vi "抓邊_new.vi"(0 "Image In":T7, 1 "Process":T10(ring), 2 "Optimized Mode":bool, 5 "ROI":T8, 7 "Options":T6={"Search Direction"=0, "Edge Options"={"Edge Polarity"=0, "Kernel Size"=3, "Width"=3, "Minimum Edge Strength"=10.0, "Interpolation Type"=enum."Bilinear Fixed", "Data Processing Method"=enum."Average"}, "Show Search Area"=FALSE, "Show Search Lines"=FALSE, "Show Edges Found"=FALSE, "Show Result"=TRUE, "Search Area Color"=65280, "Search Lines Color"=255, "Edge Locations Color"=16776960, "Result Color"=16711680, "Overlay Group Name"=""} {"Edge Options"."Edge Polarity" items=["All Edges", "Rising Edges", "Falling Edges"]; "Edge Options"."Minimum Edge Strength" format="%.2f"; "Edge Options"."Width" step=2; "Edge Options"."Kernel Size" step=2; "Search Direction" items=["Left to Right", "Right to Left", "Top to Bottom", "Bottom to Top"]}, 9 "Gap":i32=10 min=1 max=300, 11 "error In":errorcluster, 13 "Point Diameter (5)":u32=5 min=3 max=1000) -> (4 "Image Out":T7, 6 "Line Profile":T9(graph), 8 "Line Segment":T1 {"Point 2"."Y" format="%.2f"; "Point 2"."X" format="%.2f"; "Point 1"."Y" format="%.2f"; "Point 1"."X" format="%.2f"}, 10 "Gradient Information":dbl[][](graph), 14 "Line Data":cluster{"X":sgl, "Y":sgl, "T":sgl}, 15 "error out":errorcluster)   [LabVIEW 2015]
uses:
  <vilib>/vision/Image Controls.llb/IMAQ Image.ctl
  <vilib>/vision/Measure.llb/Edge Options.ctl
  <vilib>/vision/Measure.llb/Edge Polarity.ctl
  <vilib>/vision/Measure.llb/Straight Edge Options.ctl
  <vilib>/vision/Measure.llb/Straight Edge Process.ctl
  <vilib>/vision/NI_Vision_Development_Module.lvlib
panel:
  in  "Line Fit Options":T2={"Number of Lines"=1, "Type"=enum."First Edge Rake", "Min. Score"=10.0, "Max. Score"=1000.0, "Orientation"=0.0, "Angle Range"=45.0, "Angle Tolerance"=1.0, "Step Size"=7, "Min. SNR (db)"=0.0, "Min. Points (%)"=25.0, "Hough Iterations"=5} {"Min. Points (%)" min=0.0 max=100.0; "Min. SNR (db)" min=0.0; "Max. Score" min=0.0 max=1024.0; "Min. Score" min=0.0 max=1024.0 step=1.0}
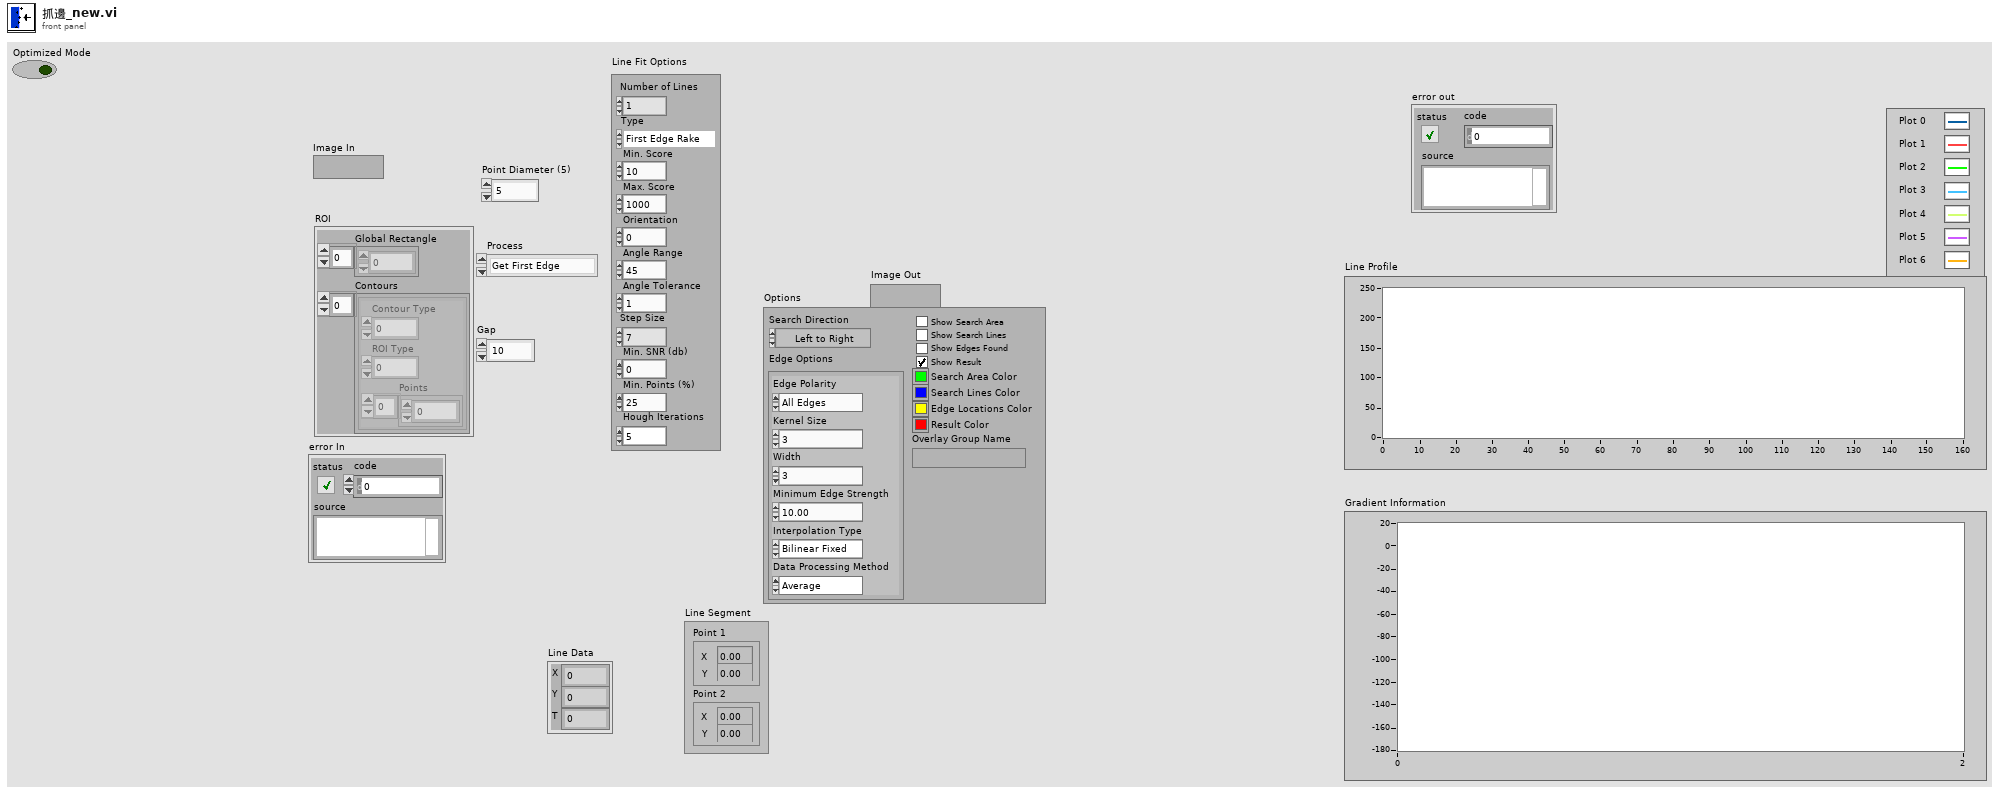
[diagram p1: front panel]
types:
  T1 = cluster{"Point 1":cluster{"X":sgl, "Y":sgl}, "Point 2":cluster{"X":sgl, "Y":sgl}}
  T2 = typedef "Straight Edge Options.ctl" = cluster{"Number of Lines":i32, "Type":T3, "Min. Score":dbl, "Max. Score":dbl, "Orientation":dbl, "Angle Range":dbl, "Angle Tolerance":dbl, "Step Size":u32, "Min. SNR (db)":dbl, "Min. Points (%)":dbl, "Hough Iterations":i32}
  T3 = typedef "Straight Edge Process.ctl" = enum32{"First Edge Rake", "Best Edge Rake", "Hough Edge Rake", "First Edge Projection", "Best Edge Projection"}
  T4 = typedef "Edge Options.ctl" = cluster{"Edge Polarity":T5, "Kernel Size":u32, "Width":u32, "Minimum Edge Strength":sgl, "Interpolation Type":enum32{"Zero Order", "Bilinear", "Quadratic", "Cubic", "Bilinear Fixed"}, "Data Processing Method":enum32{"Average", "Median"}}
  T5 = typedef "Edge Polarity.ctl" = u32
  T6 = cluster{"Search Direction":u32, "Edge Options":T4, "Show Search Area":bool, "Show Search Lines":bool, "Show Edges Found":bool, "Show Result":bool, "Search Area Color":u32, "Search Lines Color":u32, "Edge Locations Color":u32, "Result Color":u32, "Overlay Group Name":string}
  T7 = typedef "IMAQ Image.ctl" = refnum<image>
  T8 = cluster{"Global Rectangle":i32[], "Contours":cluster{"Contour Type":u32, "ROI Type":u32, "Points":i32[]}[]}
  T9 = cluster{"x0":sgl, "dx":sgl, "Pixels Line":sgl[]}[]
  T10 = enum16{"Get First Edge", "Get First + Last Edge", "Get All Edges", "Get Best Edge"}
  T11 = typedef "IMAQ Line" = cluster{"Start X":i32, "Start Y":i32, "End X":i32, "End Y":i32}
  T12 = cluster{"Point 1":cluster{"x":dbl, "y":dbl}, "Point 2":cluster{"x":dbl, "y":dbl}}
  T13 = typedef "IMAQ Rectangle" = cluster{"Left":i32, "Top":i32, "Right":i32, "Bottom":i32, "Rotation":dbl}
  T14 = typedef "IMAQ Point" = cluster{"X":sgl, "Y":sgl}
  T15 = cluster{"Left":i32, "Top":i32, "Right":i32, "Bottom":i32}
  T16 = typedef "ROI Descriptor" = cluster{"Global Rectangle":i32[], "Contours":cluster{"ID":enum32{"External", "Internal"}, "Type":u32, "Coordinates":i32[]}[]}
  T17 = typedef "Edge New.ctl" = cluster{"Location (Pixel)":cluster{"X":sgl, "Y":sgl}, "Location (Real-World)":cluster{"X":sgl, "Y":sgl}, "Distance (Pixel)":dbl, "Distance (Real-World)":dbl, "Strength":dbl, "Noise":dbl, "Rising?":bool}
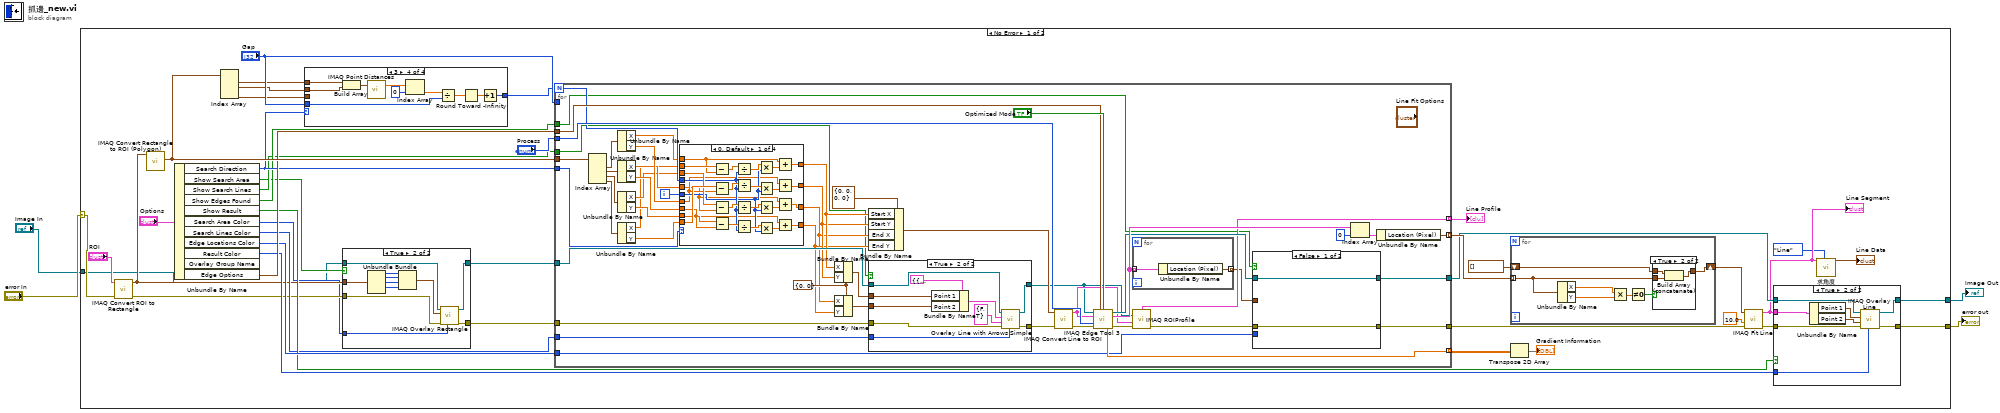
[diagram p0: block diagram]
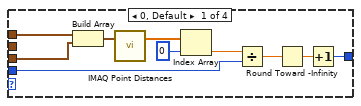
[diagram p4: hidden frame]
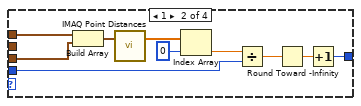
[diagram p5: hidden frame]
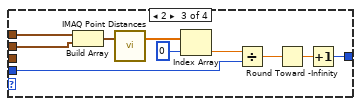
[diagram p6: hidden frame]
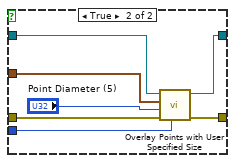
[diagram p9: hidden frame]
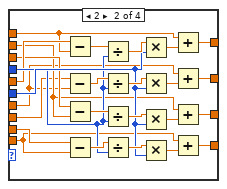
[diagram p10: hidden frame]
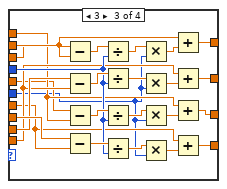
[diagram p11: hidden frame]
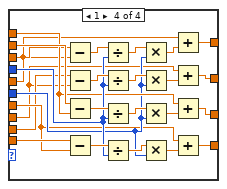
[diagram p12: hidden frame]
diagram:
  n1 = case shown="No Error" "error In" {
    selector: "error In" -> [w7 w297]
    tunnel: [w8 w297] -> w4
    tunnel: [w6 w296] -> w2
    tunnel: "Image In" -> [w5 w296]
    frame No Error {
      n2 = call "IMAQ Convert ROI to Rectangle"("error in (no error)"=w7, "ROI Descriptor"="ROI") -> ("error out"=w12:errorcluster, "Rectangle"=w13:T13)  [unwired: 7 in]
      n3 = call "IMAQ Convert Rectangle to ROI (Polygon)"("Rectangle"=w13) -> ("Rectangle Points"=w34:T14[])  [unwired: 7 in, 2 out]
      n4 = Unbundle By Name("Options") -> ("Search Direction"=w21:u32, "Show Search Area"=w10:bool, "Show Search Lines"=w16:bool, "Show Edges Found"=w19:bool, "Show Result"=w18:bool, "Search Area Color"=w9:u32, "Search Lines Color"=w15:u32, "Edge Locations Color"=w20:u32, "Result Color"=w17:u32, "Edge Options"=w22:T4)  [unwired: 1 out]
      n5 = Index Array(array=w34) -> (element #1=w32:T14, element #2=w31:T14, element #4=w30:T14)  [unwired: 4 in, 1 out]
      n6 = case shown="3" w21 {
        tunnel: "Gap" -> [w75 w85 w95 w105]
        tunnel: [w74 w84 w94 w104] -> w40
        tunnel: w32 -> [w71 w81 w93 w101]
        tunnel: w30 -> [w70 w80 _ _]
        tunnel: w31 -> [_ _ w89 w100]
        frame 0, Default {
          n7 = Build Array(w71, w70) -> (w73:T14[])
          n8 = call "IMAQ Point Distances"("Points"=w73) -> ("Distances"=w72:sgl[])  [unwired: 4 in, 1 out]
          n9 = Index Array(array=w72, index=0) -> (element=w68:sgl)
          n10 = Divide(x=w68, y=w75) -> (x/y=w76:sgl)
          n11 = Round Toward -Infinity(1:w76) -> (0:w77:sgl)
          n12 = Increment(x=w77) -> (x+1=w74:i32)
        }
        frame 1 {
          n13 = Build Array(w81, w80) -> (w83:T14[])
          n14 = call "IMAQ Point Distances"("Points"=w83) -> ("Distances"=w82:sgl[])  [unwired: 4 in, 1 out]
          n15 = Index Array(array=w82, index=0) -> (element=w78:sgl)
          n16 = Divide(x=w78, y=w85) -> (x/y=w86:sgl)
          n17 = Round Toward -Infinity(1:w86) -> (0:w87:sgl)
          n18 = Increment(x=w87) -> (x+1=w84:i32)
        }
        frame 2 {
          n19 = Build Array(w93, w89) -> (w92:T14[])
          n20 = call "IMAQ Point Distances"("Points"=w92) -> ("Distances"=w91:sgl[])  [unwired: 4 in, 1 out]
          n21 = Index Array(array=w91, index=0) -> (element=w90:sgl)
          n22 = Divide(x=w90, y=w95) -> (x/y=w96:sgl)
          n23 = Round Toward -Infinity(1:w96) -> (0:w97:sgl)
          n24 = Increment(x=w97) -> (x+1=w94:i32)
        }
        frame 3 {
          n25 = Build Array(w101, w100) -> (w103:T14[])
          n26 = call "IMAQ Point Distances"("Points"=w103) -> ("Distances"=w102:sgl[])  [unwired: 4 in, 1 out]
          n27 = Index Array(array=w102, index=0) -> (element=w99:sgl)
          n28 = Divide(x=w99, y=w105) -> (x/y=w106:sgl)
          n29 = Round Toward -Infinity(1:w106) -> (0:w107:sgl)
          n30 = Increment(x=w107) -> (x+1=w104:i32)
        }
      }
      n31 = case shown="True" w10 {
        tunnel: w5 -> [w45 w57]
        tunnel: [w45 w56] -> w14
        tunnel: w13 -> [_ w55]
        tunnel: w12 -> [w46 w49]
        tunnel: [w46 w48] -> w11
        tunnel: w9 -> [_ w47]
        frame False {
        }
        frame True {
          n32 = Unbundle(w55) -> ("Left"=w54:i32, "Top"=w53:i32, "Right"=w52:i32, "Bottom"=w51:i32)  [unwired: 1 out]
          n33 = Bundle("Left"=w54, "Top"=w53, "Right"=w52, "Bottom"=w51) -> (w50:T15)  [unwired: 1 in]
          n34 = call "IMAQ Overlay Rectangle"("Color"=w47, "error in (no error)"=w49, "Rectangle"=w50, "Image"=w57) -> ("error out"=w48:errorcluster, "Image Out"=w56:T7)  [unwired: 6 in]
        }
      }
      n35 = for {
        N: w40 -> [w154]
        tunnel: w21 -> [w152]
        tunnel: [w163] -> w37
        tunnel: w14 -> [w153]
        tunnel: w11 -> [w151]
        tunnel: [w162] -> w35
        tunnel: "Process" -> [w164]
        tunnel: w22 -> [w161]
        tunnel: [w160] -> w39 mode=indexing
        tunnel: [w159] -> w41 mode=indexing
        tunnel: [w158] -> w38 mode=indexing
        tunnel: "Gap" -> [_]
        tunnel: w34 -> [w150]
        tunnel: w20 -> [w122]
        tunnel: w19 -> [w121]
        tunnel: w16 -> [w120]
        tunnel: w15 -> [w119]
        i -> [w123]
        w147 = cluster{"X":i32, "Y":i32} {"X"=0, "Y"=0} ("Start Point")
        n36 = Index Array(array=w150) -> (element #1=w135:T14, element #2=w134:T14, element #3=w133:T14, element #4=w132:T14)  [unwired: 4 in]
        n37 = Unbundle By Name(w135) -> ("X"=w131:sgl, "Y"=w130:sgl)
        n38 = Unbundle By Name(w134) -> ("X"=w129:sgl, "Y"=w128:sgl)
        n39 = Unbundle By Name(w133) -> ("X"=w127:sgl, "Y"=w126:sgl)
        n40 = Unbundle By Name(w132) -> ("X"=w125:sgl, "Y"=w124:sgl)
        n41 = case shown="0, Default" w152 {
          tunnel: [w200 w219 w245 w270] -> w142
          tunnel: [w195 w218 w244 w271] -> w139
          tunnel: [w198 w216 w242 w268] -> w141
          tunnel: [w194 w217 w243 w269] -> w140
          tunnel: w125 -> [w213 w224 w250 w280]
          tunnel: w131 -> [w191 w226 w249 w279]
          tunnel: w154 -> [w204 w228 w255 w281]
          tunnel: w123 -> [w203 w229 w246 w278]
          tunnel: w124 -> [w210 w220 w252 w275]
          tunnel: w130 -> [w193 w222 w251 w274]
          tunnel: w127 -> [w207 w225 w248 w277]
          tunnel: w129 -> [w192 w227 w247 w276]
          tunnel: w126 -> [w202 w221 w253 w273]
          tunnel: w128 -> [w190 w223 w254 w272]
          frame 0, Default {
            n42 = Subtract(x=w213, y=w191) -> (x-y=w214:sgl)
            n43 = Subtract(x=w210, y=w193) -> (x-y=w212:sgl)
            n44 = Subtract(x=w207, y=w192) -> (x-y=w209:sgl)
            n45 = Subtract(x=w202, y=w190) -> (x-y=w205:sgl)
            n46 = Divide(x=w214, y=w204) -> (x/y=w215:sgl)
            n47 = Divide(x=w212, y=w204) -> (x/y=w211:sgl)
            n48 = Divide(x=w209, y=w204) -> (x/y=w208:sgl)
            n49 = Divide(x=w205, y=w204) -> (x/y=w206:sgl)
            n50 = Multiply(x=w215, y=w203) -> (x*y=w201:sgl)
            n51 = Multiply(x=w211, y=w203) -> (x*y=w199:sgl)
            n52 = Multiply(x=w208, y=w203) -> (x*y=w197:sgl)
            n53 = Multiply(x=w206, y=w203) -> (x*y=w196:sgl)
            n54 = Add(x=w191, y=w201) -> (x+y=w200:sgl)
            n55 = Add(x=w193, y=w199) -> (x+y=w198:sgl)
            n56 = Add(x=w192, y=w197) -> (x+y=w195:sgl)
            n57 = Add(x=w190, y=w196) -> (x+y=w194:sgl)
          }
          frame 2 {
            n58 = Subtract(x=w227, y=w226) -> (x-y=w240:sgl)
            n59 = Subtract(x=w223, y=w222) -> (x-y=w239:sgl)
            n60 = Subtract(x=w225, y=w224) -> (x-y=w237:sgl)
            n61 = Subtract(x=w221, y=w220) -> (x-y=w234:sgl)
            n62 = Divide(x=w240, y=w228) -> (x/y=w241:sgl)
            n63 = Divide(x=w239, y=w228) -> (x/y=w238:sgl)
            n64 = Divide(x=w237, y=w228) -> (x/y=w236:sgl)
            n65 = Divide(x=w234, y=w228) -> (x/y=w235:sgl)
            n66 = Multiply(x=w241, y=w229) -> (x*y=w233:sgl)
            n67 = Multiply(x=w238, y=w229) -> (x*y=w232:sgl)
            n68 = Multiply(x=w236, y=w229) -> (x*y=w231:sgl)
            n69 = Multiply(x=w235, y=w229) -> (x*y=w230:sgl)
            n70 = Add(x=w226, y=w233) -> (x+y=w219:sgl)
            n71 = Add(x=w222, y=w232) -> (x+y=w216:sgl)
            n72 = Add(x=w224, y=w231) -> (x+y=w218:sgl)
            n73 = Add(x=w220, y=w230) -> (x+y=w217:sgl)
          }
          frame 3 {
            n74 = Subtract(x=w248, y=w250) -> (x-y=w263:sgl)
            n75 = Subtract(x=w253, y=w252) -> (x-y=w260:sgl)
            n76 = Subtract(x=w247, y=w249) -> (x-y=w266:sgl)
            n77 = Subtract(x=w254, y=w251) -> (x-y=w265:sgl)
            n78 = Divide(x=w263, y=w255) -> (x/y=w262:sgl)
            n79 = Divide(x=w260, y=w255) -> (x/y=w261:sgl)
            n80 = Divide(x=w266, y=w255) -> (x/y=w267:sgl)
            n81 = Divide(x=w265, y=w255) -> (x/y=w264:sgl)
            n82 = Multiply(x=w262, y=w246) -> (x*y=w257:sgl)
            n83 = Multiply(x=w261, y=w246) -> (x*y=w256:sgl)
            n84 = Multiply(x=w267, y=w246) -> (x*y=w259:sgl)
            n85 = Multiply(x=w264, y=w246) -> (x*y=w258:sgl)
            n86 = Add(x=w250, y=w257) -> (x+y=w245:sgl)
            n87 = Add(x=w252, y=w256) -> (x+y=w242:sgl)
            n88 = Add(x=w249, y=w259) -> (x+y=w244:sgl)
            n89 = Add(x=w251, y=w258) -> (x+y=w243:sgl)
          }
          frame 1 {
            n90 = Subtract(x=w277, y=w276) -> (x-y=w289:sgl)
            n91 = Subtract(x=w273, y=w272) -> (x-y=w286:sgl)
            n92 = Subtract(x=w280, y=w279) -> (x-y=w292:sgl)
            n93 = Subtract(x=w275, y=w274) -> (x-y=w291:sgl)
            n94 = Divide(x=w289, y=w281) -> (x/y=w288:sgl)
            n95 = Divide(x=w286, y=w281) -> (x/y=w287:sgl)
            n96 = Divide(x=w292, y=w281) -> (x/y=w293:sgl)
            n97 = Divide(x=w291, y=w281) -> (x/y=w290:sgl)
            n98 = Multiply(x=w288, y=w278) -> (x*y=w283:sgl)
            n99 = Multiply(x=w287, y=w278) -> (x*y=w282:sgl)
            n100 = Multiply(x=w293, y=w278) -> (x*y=w285:sgl)
            n101 = Multiply(x=w290, y=w278) -> (x*y=w284:sgl)
            n102 = Add(x=w276, y=w283) -> (x+y=w270:sgl)
            n103 = Add(x=w272, y=w282) -> (x+y=w268:sgl)
            n104 = Add(x=w279, y=w285) -> (x+y=w271:sgl)
            n105 = Add(x=w274, y=w284) -> (x+y=w269:sgl)
          }
        }
        n106 = Bundle By Name(cluster=w147, "X"=w142, "Y"=w141) -> (w145:cluster{"X":i32, "Y":i32})
        n107 = Bundle By Name(cluster=w147, "X"=w139, "Y"=w140) -> (w146:cluster{"X":i32, "Y":i32})
        n108 = Bundle By Name(cluster=T11 {"Start X"=0, "Start Y"=0, "End X"=0, "End Y"=0} ("Line"), "Start X"=w142, "Start Y"=w141, "End X"=w139, "End Y"=w140) -> (w148:T11)
        n109 = case shown="True" w120 {
          tunnel: w153 -> [w170 w180]
          tunnel: w151 -> [w169 w179]
          tunnel: w146 -> [_ w178]
          tunnel: w145 -> [_ w177]
          tunnel: [w170 w173] -> w144
          tunnel: [w169 w172] -> w143
          tunnel: w119 -> [_ w171]
          frame False {
          }
          frame True {
            n110 = Bundle By Name(cluster=T12 {"Point 1"={"x"=50.0, "y"=50.0}, "Point 2"={"x"=70.0, "y"=70.0}} ("Line Coordinates"), "Point 1"=w177, "Point 2"=w178) -> (w174:T12)
            n111 = call "Overlay Line with Arrows Simple.vi"("Color"=w171, "error in"=w179, "Arrows"=cluster{"Start point":bool, "End point":bool} {"Start point"=FALSE, "End point"=TRUE}, "Line Coordinates"=w174, "Image In"=w180) -> ("error out"=w172:errorcluster, "Image Out"=w173:T7)  [unwired: 5 in]
          }
        }
        n112 = call "IMAQ Convert Line to ROI"("error in (no error)"=w143, "Line"=w148) -> ("error out"=w156:errorcluster, "ROI Descriptor"=w155:T16)  [unwired: 7 in]
        n113 = call "IMAQ Edge Tool 3"("Image"=w144, "Edge Options"=w161, "Optimized Mode"="Optimized Mode", "ROI Descriptor"=w155, "Process"=w164, "error in (no error)"=w156) -> ("Image (duplicate)"=w165:T7, "Edge Information"=w168:T17[], "Gradient Values"=w159:dbl[], "error out"=w157:errorcluster)  [unwired: 5 in, 1 out]
        n114 = for {
          tunnel: w168 -> [w295] mode=indexing
          tunnel: [w294] -> w136 mode=indexing
          n115 = Unbundle By Name(w295) -> ("Location (Pixel)"=w294:cluster{"X":sgl, "Y":sgl})
        }
        n116 = call "IMAQ ROIProfile"("error in (no error)"=w157, "ROI Descriptor"=w155, "Image"=w144) -> ("error out"=w167:errorcluster, "ROI Graph"=w160:cluster{"x0":sgl, "dx":sgl, "Pixels Line":sgl[]})  [unwired: 1 in, 3 out]
        n117 = case shown="False" w121 {
          tunnel: w167 -> [w181 w189]
          tunnel: w165 -> [w182 w188]
          tunnel: [w182 w187] -> w163
          tunnel: [w181 w186] -> w162
          tunnel: w136 -> [_ w185]
          tunnel: w122 -> [_ w183]
          frame False {
          }
          frame True {
            n118 = call "Overlay Points with User Specified Size.vi"("Color"=w183, "error in"=w189, "Point Diameter (5)"="Point Diameter (5)", "Points"=w185, "Image In"=w188) -> ("error out"=w186:errorcluster, "Image Out"=w187:T7)  [unwired: 5 in]
          }
        }
        n119 = Index Array(array=w168, index=0) -> (element=w137:T17)
        n120 = Unbundle By Name(w137) -> ("Location (Pixel)"=w158:cluster{"X":sgl, "Y":sgl})
      }
      "Line Profile" <- w39
      n121 = for {
        tunnel: w38 -> [w110] mode=indexing
        shift-right: [w109] -> w36
        shift-left: cluster{"X":sgl, "Y":sgl}[] [] -> [w108]
        n122 = Unbundle By Name(w110) -> ("X"=w114:sgl, "Y"=w113:sgl)
        n123 = Multiply(x=w114, y=w113) -> (x*y=w112:sgl)
        n124 = Not Equal To 0?(x=w112) -> (x != 0?=w111:bool)
        n125 = case shown="True" w111 {
          tunnel: w110 -> [_ w118]
          tunnel: [w115 w117] -> w109
          tunnel: w108 -> [w115 w116]
          frame False {
          }
          frame True {
            n126 = Build Array (concatenate)(w116, w118) -> (w117:cluster{"X":sgl, "Y":sgl}[])
          }
        }
      }
      n127 = Transpose 2D Array(2D array=w41) -> (transposed array=→"Gradient Information":dbl[][])
      n128 = call "IMAQ Fit Line"("error in (no error)"=w35, "Pixel Radius"=sgl 10.0, "Points"=w36) -> ("error out"=w28:errorcluster, "Line Segment"=w26:T1)  [unwired: 3 in, 4 out]
      "Line Segment" <- w26
      n129 = case shown="True" w18 {
        tunnel: w37 -> [w59 w67]
        tunnel: [w58 w66] -> w8
        tunnel: w28 -> [w58 w63]
        tunnel: w26 -> [_ w62]
        tunnel: [w59 w61] -> w6
        tunnel: w17 -> [_ w60]
        frame False {
        }
        frame True {
          n130 = Unbundle By Name(w62) -> ("Point 1"=w64:cluster{"X":sgl, "Y":sgl}, "Point 2"=w65:cluster{"X":sgl, "Y":sgl})
          n131 = call "IMAQ Overlay Line"("Color"=w60, "error in (no error)"=w63, "End Point"=w65, "Start Point"=w64, "Image"=w67) -> ("error out"=w66:errorcluster, "Image Out"=w61:T7)  [unwired: 5 in]
        }
      }
      n132 = call "求角度.vi"("Line form"=enum16{"Line", "Two Point"}."Line", "Line"=w26) -> ("Line Data"=→"Line Data":cluster{"X":sgl, "Y":sgl, "T":sgl})  [unwired: 9 in]
    }
    frame Error {
    }
  }
  "error out" <- w4
  "Image Out" <- w2
